vi "Stop Drawing.vi"(8 "error in (no error)":errorcluster, 11 "Field Drawer in":refnum<class "Field Drawer.lvclass">) -> (0 "error out":errorcluster, 3 "Field Drawer out":refnum<class "Field Drawer.lvclass">)   [LabVIEW 2022 SP3, in "Vision.lvlib" / "Field Drawer.lvlib" / "Field Drawer.lvclass"]
uses:
  Field Drawer.lvclass
  Field Drawer.lvclass/Field Drawer.ctl
  Old vision/Controls/Field Size.ctl
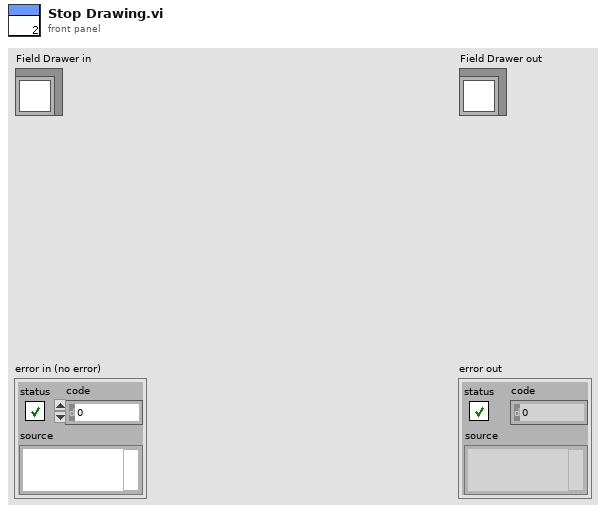
[diagram p1: front panel]
types:
  T1 = typedef "Field Size.ctl" = cluster{"line_width":u32, "field_length":u32, "field_width":u32, "boundary_width":u32, "referee_width":u32, "goal_width":u32, "goal_depth":u32, "goal_wall_width":u32, "center_circle_radius":u32, "defense_radius":u32, "defense_stretch":u32, "free_kick_from_defense_dist":u32, "penalty_spot_from_field_line_dist":u32, "penalty_line_from_spot_dist":u32}
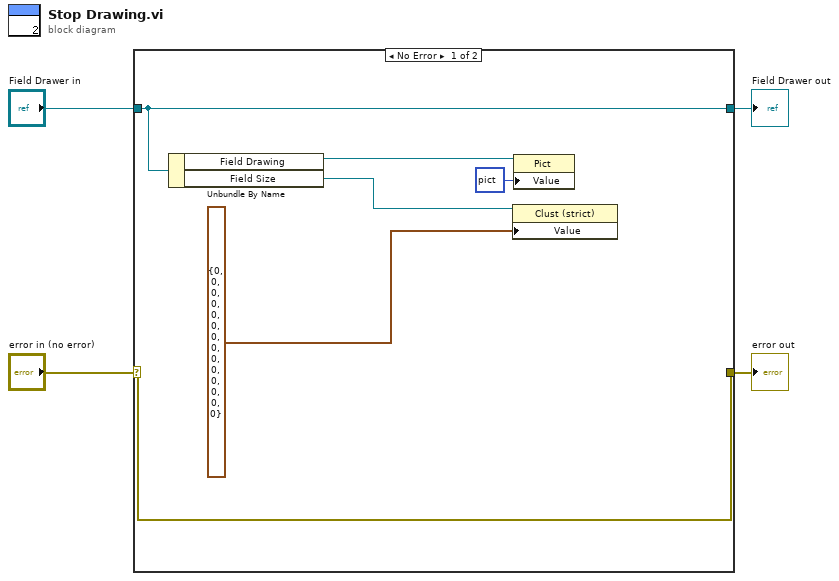
[diagram p0: block diagram]
diagram:
  n1 = case shown="No Error" "error in (no error)" {
    selector: "error in (no error)" -> [w10 w12]
    tunnel: [w10 w12] -> w3
    tunnel: [w9 w11] -> w1
    tunnel: "Field Drawer in" -> [w9 w11]
    frame No Error {
      n2 = Unbundle By Name(w9) -> ("Field Drawing"=w8:refnum<vi>, "Field Size"=w7:refnum<vi>)
      n3 = property class="Clust (strict)"(reference=w7, "Value"=T1 {"line_width"=0, "field_length"=0, "field_width"=0, "boundary_width"=0, "referee_width"=0, "goal_width"=0, "goal_depth"=0, "goal_wall_width"=0, "center_circle_radius"=0, "defense_radius"=0, "defense_stretch"=0, "free_kick_from_defense_dist"=0, "penalty_spot_from_field_line_dist"=0, "penalty_line_from_spot_dist"=0}) -> ()  [unwired: 1 in, 2 out]
      n4 = property class="Pict"(reference=w8, "Value"=picture data[5B]) -> ()  [unwired: 1 in, 2 out]
    }
    frame Error {
    }
  }
  "error out" <- w3
  "Field Drawer out" <- w1
